vi "AIsFIFORT.vi"(1 "P0":dbl[](array[numeric]), 2 "P1":dbl[](array[numeric]), 3 "P2":dbl[](array[numeric]), 4 "FPGA VI Reference In":refnum<k20>) -> ()   [LabVIEW 2010]
uses:
  <vilib>/rvi/interface/nirviMethod/nirviMethod.xnode
  C:/Users/HAGAR-IV/Desktop/Zeugs/markus/version feb 2012/FPGA Bitfiles/pertrasgcfpga2_FPGATarget_FPGA-Programm-10_16368CB6.lvbitx
  C:/Users/HAGAR-IV/Desktop/Zeugs/Johnny/pertrasgc fpga/FPGA-Programm-10-14.vi
  <vilib>/rvi/interface/common/niFpgaNodeNameForErrorReporting.ctl
  <vilib>/rvi/errors/niLvFpgaWhatHappensToTopLevelVI.ctl
  <vilib>/rvi/interface/nirviReadWriteControl/nirviReadWriteControl.xnode
  GVAIs.vi
  gvbooleschRT.vi
  <vilib>/Utility/error.llb/Error Cluster From Error Code.vi
  <vilib>/rvi/errors/niLvFpgaAdjustHostInterfaceError.vi
  NiFpgaLv.dll
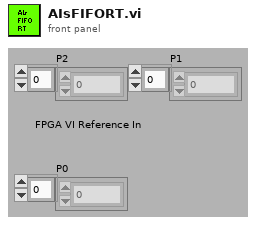
[diagram p1: front panel]
types:
  T1 = typedef "niFpgaNodeNameForErrorReporting.ctl" = enum16{"Open FPGA VI Reference", "Read/Write Control", "Invoke Method: Abort", "Invoke Method: Acknowledge IRQ", "Invoke Method: Download", "Invoke Method: FIFO.Configure", "Invoke Method: FIFO.Read", "Invoke Method: FIFO.Start", "Invoke Method: FIFO.Stop", "Invoke Method: FIFO.Write", "Invoke Method: Reset", "Invoke Method: Run", "Invoke Method: Wait on IRQ", "Close FPGA VI Reference"}
  T2 = typedef "niLvFpgaWhatHappensToTopLevelVI.ctl" = enum16{"top level VI scripted behind XNode", "top level VI inlined behind XNode"}
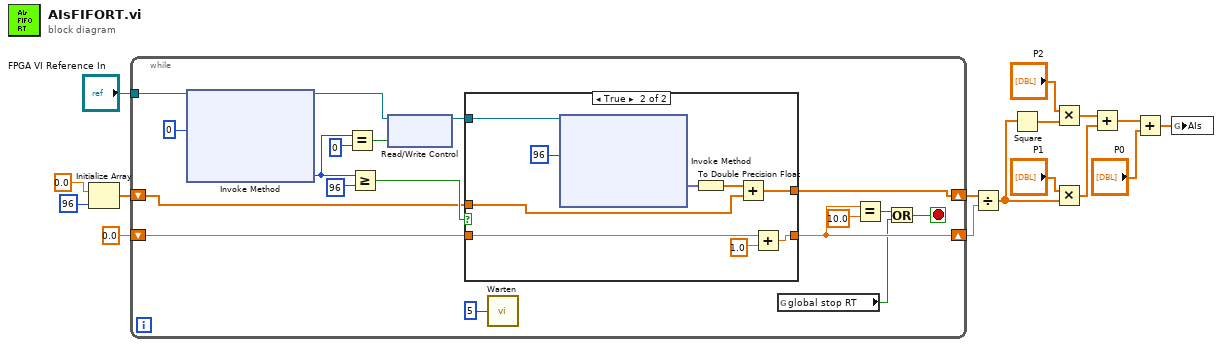
[diagram p0: block diagram]
diagram:
  n1 = Initialize Array(0.0 ("Element"), 96 ("Dimension")) -> (w3:dbl[])
  n2 = while {
    tunnel: "FPGA VI Reference In" -> [w34]
    shift-right: [w28] -> w15
    shift-left: w3 -> [w29]
    shift-right: [w26] -> w2
    shift-left: 0.0 -> [w27]
    stop <- w19 stop-if-true
    n3 = xnode "Invoke Method"("FPGA VI Reference In"=w34, "Number of Elements"=u32 0) -> ("FPGA VI Reference Out"=w17:refnum<k20>, "Elements Remaining"=w24:u32)  [unwired: 2 in, 2 out]
    n4 = Equal?(x=w24, y=u32 0) -> (x = y?=w22:bool)
    n5 = Greater Or Equal?(x=w24, y=u32 96) -> (x >= y?=w31:bool)
    n6 = xnode "Read/Write Control"("FPGA VI Reference In"=w17, "FIFO leer"=w22) -> ("FPGA VI Reference Out"=w18:refnum<k20>)  [unwired: 1 in, 1 out]
    n7 = case shown="True" w31 {
      tunnel: w18 -> [_ w155]
      tunnel: w29 -> [w146 w151]
      tunnel: [w146 w150] -> w28
      tunnel: w27 -> [w145 w149]
      tunnel: [w145 w147] -> w26
      frame False {
      }
      frame True {
        n8 = xnode "Invoke Method"("FPGA VI Reference In"=w155, "Number of Elements"=u32 96) -> ("Data"=w153:fxp<+/-,26,5>[])  [unwired: 2 in, 3 out]
        n9 = To Double Precision Float(number=w153) -> (double precision float=w152:dbl[])
        n10 = Add(x=w152, y=w151) -> (x+y=w150:dbl[])
        n11 = Add(x=w149, y=1.0) -> (x+y=w147:dbl)
      }
    }
    n12 = call "Warten"("Count(mSec)"=u32 5) -> ()  [unwired: 1 out]
    n13 = global read "gvbooleschRT.vi" "global stop RT"() -> (w21:bool)
    n14 = Equal?(x=w26, y=10.0) -> (x = y?=w20:bool)
    n15 = Or(x=w20, y=w21) -> (x .or. y?=w19:bool)
  }
  n16 = Divide(x=w15, y=w2) -> (x/y=w10:dbl[])
  n17 = Square(x=w10) -> (x^2=w13:dbl[])
  n18 = Multiply(x="P2", y=w13) -> (x*y=w9:dbl[])
  n19 = Multiply(x="P1", y=w10) -> (x*y=w8:dbl[])
  n20 = Add(x=w9, y=w8) -> (x+y=w7:dbl[])
  n21 = Add(x=w7, y="P0") -> (x+y=w1:dbl[])
  n22 = global write "GVAIs.vi" "AIs"(w1) -> ()
